vi "LVClass_SlopesPostProcessList ctor.vi"(0 "SlopesPostProcessorList (const)":refnum<class "SlopesPostProcessorList.lvclass">, 5 "Dimensions_um":T1={"Size"={"X"=32, "Y"=32}, "Step"={"X"=1.0, "Y"=1.0}}, 7 "serial":string="7102", 11 "error in (no error)":errorcluster) -> (4 "SlopesPostProcessorList (new)":refnum<class "SlopesPostProcessorList.lvclass">, 15 "error out":errorcluster)   [LabVIEW 2020, in "SlopesPostProcessorList.lvclass"]
doc: "SlopesPostProcessorList default constructor.\n\n--------------------------------------------------------------------------------\n\n<B>SlopesPostProcessorListIn </B> : Constant Pointer to SlopesPostProcessorList object.\n<B>SlopesPostProcessorListOut </B> : Constant Pointer to SlopesPostProcessorList object.\n<B>ErrorIn </B> : Error\n<B>ErrorOut </B> : Error\n\n--------------------------------------------------------------------------------"
uses:
  SlopesPostProcessorList.lvclass
  Controls/General dimensions definition.ctl
  Controls/Point2D.ctl
  Controls/Point2Df.ctl
  Controls/Handle creation.ctl
  SlopesPostProcessorList.lvclass/SlopesPostProcessorList.ctl
  HasoSlopes/HasoSlopes.lvclass
  Pupil/Pupil.lvclass
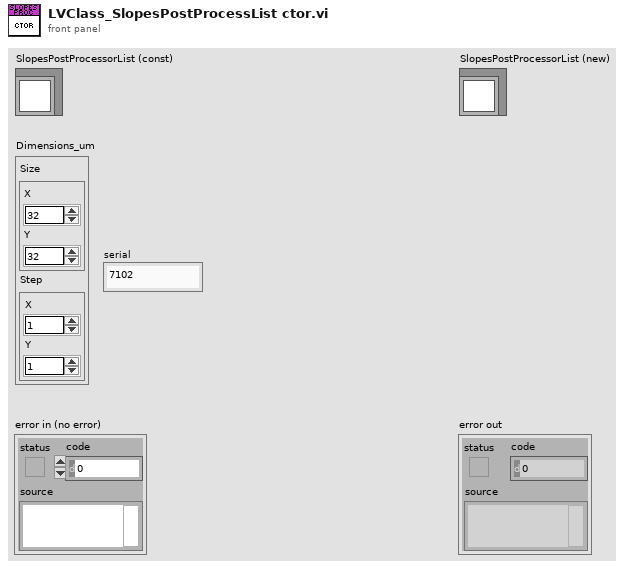
[diagram p1: front panel]
types:
  T1 = typedef "General dimensions definition.ctl" = cluster{"Size":T2, "Step":T3}
  T2 = typedef "Point2D.ctl" = cluster{"X":u32, "Y":u32}
  T3 = typedef "Point2Df.ctl" = cluster{"X":sgl, "Y":sgl}
  T4 = typedef "Handle creation.ctl" = enum16{"By ctor", "By write function"}
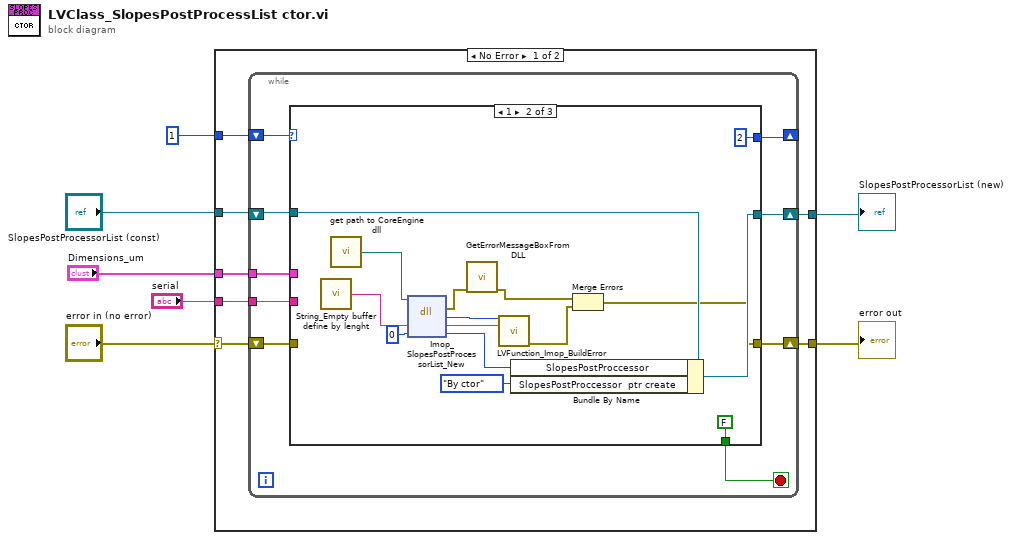
[diagram p0: block diagram]
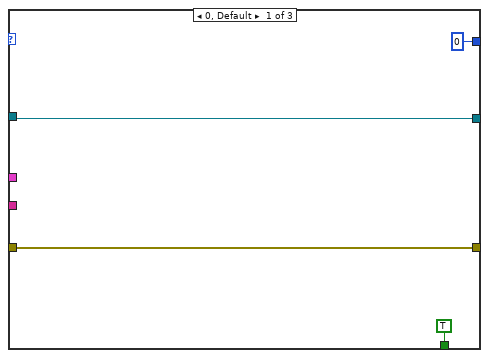
[diagram p2: hidden frame]
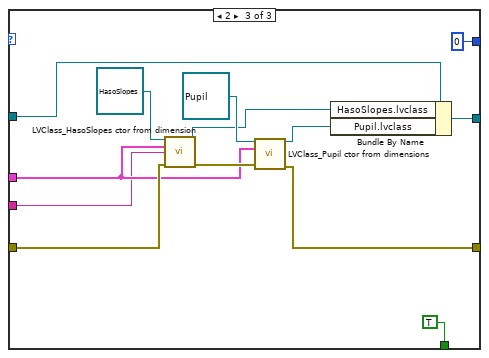
[diagram p3: hidden frame]
diagram:
  n1 = case shown="No Error" "error in (no error)" {
    selector: "error in (no error)" -> [w10 w56]
    tunnel: "SlopesPostProcessorList (const)" -> [w12 w57]
    tunnel: [w14 w57] -> w5
    tunnel: [w13 w56] -> w4
    tunnel: 1 -> [w11 _]
    tunnel: "Dimensions_um" -> [w9 _]
    tunnel: "serial" -> [w8 _]
    frame No Error {
      n2 = while {
        shift-right: [w19] -> _
        shift-left: w11 -> [w20]
        shift-right: [w22] -> w13
        shift-left: w10 -> [w18]
        shift-right: [w23] -> w14
        shift-left: w12 -> [w21]
        tunnel: w9 -> [w16]
        tunnel: w8 -> [w15]
        stop <- w17 stop-if-true
        n3 = case shown="1" w20 {
          tunnel: [w25 w38 w47] -> w23
          tunnel: [w26 w28 w51] -> w22
          tunnel: w21 -> [w25 w37 w50]
          tunnel: [0 2 0] -> w19
          tunnel: w18 -> [w26 _ w54]
          tunnel: [TRUE FALSE TRUE] -> w17
          tunnel: w16 -> [_ _ w44]
          tunnel: w15 -> [_ _ w43]
          frame 0, Default {
          }
          frame 1 {
            n4 = call "String_Empty buffer define by lenght.vi"() -> ("Empty buffer"=w42:string)  [unwired: 1 in]
            n5 = call "get path to CoreEngine dll.vi"() -> ("path to wavekit library"=w33:path)  [unwired: 14 in, 1 out]
            n6 = dll-call lib="D:/soft/HASO_v3/SVN_trunk/ImOpCoreEngine4_LV2011/DLLs/c_interface_vc100.dll" fn="Imop_SlopesPostProcessorList_New"(path in=w33, "message"=w42, "objet"=0) -> (error out=w36:errorcluster, "return type"=w39:i32, "message"=w40:string, "objet"=w41:i64)  [unwired: 2 in, 1 out]
            n7 = call "GetErrorMessageBoxFromDLL.vi"("error IN"=w36) -> ("error OUT"=w30:errorcluster)  [unwired: 10 in]
            n8 = call "LVFunction_Imop_BuildError.vi"("code"=w39, "String to Prepend to source (\"\")"=w40) -> ("error out"=w29:errorcluster)  [unwired: 13 in]
            n9 = Bundle By Name(cluster=w37, "SlopesPostProccessor"=w41, "SlopesPostProccessor  ptr create"=Handle_creation."By ctor" ("Slopes PP  ptr create")) -> (w38:refnum<class "SlopesPostProcessorList.lvclass">)
            n10 = Merge Errors(w30, w29) -> (w28:errorcluster)
          }
          frame 2 {
            n11 = call "LVClass_HasoSlopes ctor from dimension.vi"("HasoSlopes (const)"=refnum<class "HasoSlopes.lvclass"> refnum ("HasoSlopes in"), "Dimensions_um"=w44, "serial"=w43, "error in (no error)"=w54) -> ("HasoSlopes (new)"=w49:refnum<class "HasoSlopes.lvclass">, "error out"=w53:errorcluster)  [unwired: 10 in]
            n12 = call "LVClass_Pupil ctor from dimensions.vi"("Pupil (const)"=refnum<class "Pupil.lvclass"> refnum ("Pupil in"), "Dimensions_um"=w44, "error in (no error)"=w53) -> ("Pupil (new)"=w48:refnum<class "Pupil.lvclass">, "error out"=w51:errorcluster)  [unwired: 11 in]
            n13 = Bundle By Name(cluster=w50, "HasoSlopes.lvclass"=w49, "Pupil.lvclass"=w48) -> (w47:refnum<class "SlopesPostProcessorList.lvclass">)
          }
        }
      }
    }
    frame Error {
    }
  }
  "error out" <- w4
  "SlopesPostProcessorList (new)" <- w5
